vi "Get DIO Bits For Jog Mode Status.vi"(4 "error in (no error)":errorcluster, 6 "Axis (1)":i32=1 min=1 max=3, 7 "VISA resource name":refnum<visa-resource-name>) -> (0 "error out":errorcluster, 2 "DIO Bits Status For Jog Mode":bool, 3 "VISA resource name out":refnum<visa-resource-name>)   [LabVIEW 2018, in "Newport ESP301.lvlib"]
doc: "Reads the status (disable or enable) of jog through DIO bits."
uses:
  Newport ESP301.lvlib
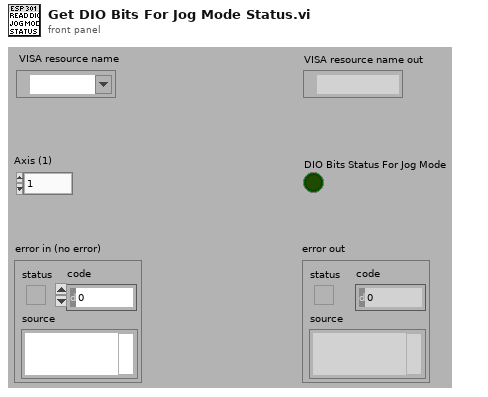
[diagram p1: front panel]
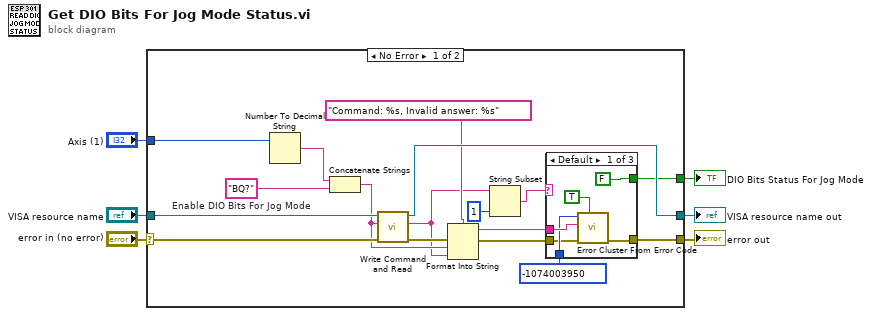
[diagram p0: block diagram]
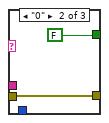
[diagram p2: hidden frame]
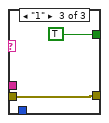
[diagram p3: hidden frame]
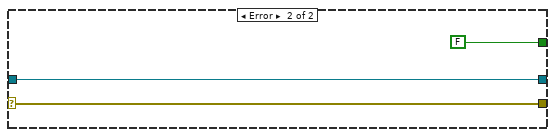
[diagram p4: hidden frame]
diagram:
  n1 = case shown="No Error" "error in (no error)" {
    selector: "error in (no error)" -> [w22 w36]
    tunnel: [w16 w36] -> w6
    tunnel: "VISA resource name" -> [w23 w35]
    tunnel: [w21 w35] -> w5
    tunnel: "Axis (1)" -> [w18 _]
    tunnel: [w10 FALSE ("Motion Done")] -> w1
    frame No Error {
      w19 = "BQ?"  # Enable DIO Bits For Jog Mode
      n2 = Number To Decimal String(number=w18) -> (decimal integer string=w20:string)  [unwired: 1 in]
      n3 = Concatenate Strings(w20, w19) -> (w11:string)
      n4 = call "Write Command and Read.vi"("error in (no error)"=w22, "Command"=w11, "VISA resource name"=w23) -> ("error out"=w15:errorcluster, "Returned string"=w8:string, "VISA resource name out"=w21:refnum<visa-resource-name>)  [unwired: 4 in]
      n5 = Format Into String(format string="Command: %s, Invalid answer: %s" ("error message (\"\")"), error in=w15, w11, w8) -> (resulting string=w17:string, error out=w14:errorcluster)  [unwired: 1 in]
      n6 = String Subset(string=w8, length (rest)=1 ("longueur (reste)")) -> (substring=w7:string)  [unwired: 1 in]
      n7 = case shown="Default" w7 {
        tunnel: [FALSE ("Motion Done") FALSE ("Motion Done") TRUE ("Motion Done")] -> w10
        tunnel: w17 -> [w27 _ _]
        tunnel: -1074003950 ("error code (0)") -> [w26 _ _]
        tunnel: w14 -> [w25 w30 w32]
        tunnel: [w24 w30 w32] -> w16
        frame Default {
          n8 = call <vilib>:"Error Cluster From Error Code.vi"("show call chain? (False)"=TRUE, "error in (no error)"=w25, "error message (\"\")"=w27, "error code (0)"=w26) -> ("error out"=w24:errorcluster)  [unwired: 5 in]
        }
        frame "0" {
        }
        frame "1" {
        }
      }
    }
    frame Error {
    }
  }
  "error out" <- w6
  "VISA resource name out" <- w5
  "DIO Bits Status For Jog Mode" <- w1
